vi "Process.vi"(8 "error in":errorcluster, 11 "Inst.Transport in":refnum<class "Inst.Transport.lvclass">) -> (0 "error out":errorcluster, 3 "Inst.Transport out":refnum<class "Inst.Transport.lvclass">)   [LabVIEW 2019, in "Inst.Transport.lvclass"]
doc: "---------------------------------------------------------------\nJKI State Machine Objects™\nhttp://jki.net/state-machine-objects/\nCopyright (C) 2005-2015, JKI <info@jki.net>\nALL RIGHTS RESERVED"
uses:
  Inst.Transport.lvclass
  <userlib>/LevyLab/Instrument Framework/Instrument/Instrument.lvclass
  <userlib>/LevyLab/RemoteControl/RemoteControl/Typedefs/Message--Cluster.ctl
  <userlib>/LevyLab/RemoteControl/RemoteControl/RemoteControl.lvclass
  Typedefs/PrivateEvents--MessageToProcess.ctl
  <userlib>/LevyLab/Debug/Debug.lvlib
  <vilib>/JKI/JKI SMO/SMO/SMO.lvclass
  Control Experiment/Control Experiment.lvclass
  Transport/Transport.lvclass
  <userlib>/LevyLab/Lockin-Multichannel/Instrument.DAQ/Typedefs/Sweep.Pattern--Enum.ctl
  <userlib>/LevyLab/Lockin-Multichannel/Instrument.DAQ/Instrument.DAQ.lvclass
  <userlib>/LevyLab/Lockin-Multichannel/Instrument.DAQ/Typedefs/Sweep.Channel--Cluster.ctl
  <userlib>/LevyLab/Lockin-Multichannel/Instrument.DAQ/Typedefs/Sweep.Channel--Cluster--Array.ctl
  Transport/Typedefs/Lockin_Sweep JSON--Cluster.ctl
  Typedefs/Inst.Transport.PublicCommands--Enum.ctl
  Typedefs/Inst.Transport.Methods--Enum.ctl
  Typedefs/startTransport--Request--Cluster.ctl
  <userlib>/LevyLab/Instrument Framework/Instrument/API/Instrument.sendMessageToProcess (variant).vi
  <userlib>/LevyLab/Instrument Framework/Instrument Types/SCPI/Instrument.SCPI.lvclass
  Typedefs/Inst.Transport.ProtectedCommands--Enum.ctl
  Typedefs/Inst.Transport.Status--Enum.ctl
  Typedefs/UI State--enum.ctl
  C:/Program Files (x86)/National Instruments/LabVIEW 2019/user.lib/LevyLab/Instrument Framework/Instrument Types/SCPI/Instrument.SCPI.lvclass
  C:/Program Files (x86)/National Instruments/LabVIEW 2019/user.lib/LevyLab/Instrument Framework/Instrument/Instrument.lvclass
  C:/Program Files (x86)/National Instruments/LabVIEW 2019/vi.lib/JKI/JKI SMO/SMO/SMO.lvclass
  Typedefs/RefreshTime--Request--Cluster.ctl
  db7760a1-0849-494e-b918-bfd2b1278472.vi
  48eb5b5f-56a5-4c0e-b192-c05c3e35427f.vi
  1045582e-a15c-4059-9878-8d398bb7fea9.vi
  8f0a8fc2-545a-492d-a380-fe326c3f5926.vi
panel:
  in  "Tab Control":enum32{"Main", "Debug"}(tab)
  in  "stopTransport":bool
  out "Status":string
  in  "Close VI":bool
  in  "Open VI":bool
  in  "Ring":u16(ring)
  out "state history":string
  out "parameters":string
  out "command":string
  out "Secret Status":string
  # "Transport Server"
  # "Inst.Transport"
  # "For instructions on how to use the JKI State Machine Objects, examples and video tutorials, visit:\nhttp://jki.net/state-machine-objects/\n\nJKI State Machine Objects™\nhttp://jki.net/state-machine-objects/\nCopyright (C) 2005-2015, JKI <info@jki.net>\nALL RIGHTS RESERVED"
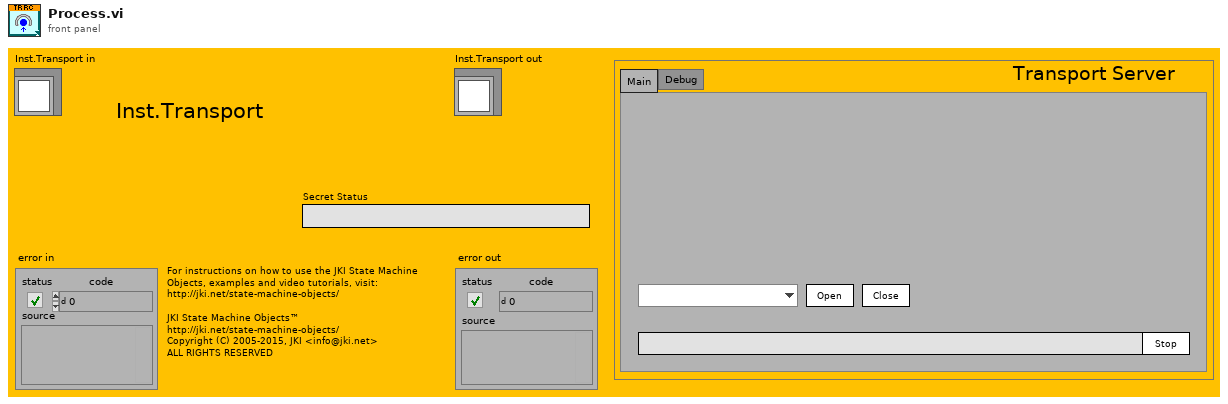
[diagram p1: front panel]
types:
  T1 = typedef "Inst.Transport.lvclass/UI State--enum.ctl" = enum16{"unknown", "Opened", "Closed"}
  T2 = typedef "Inst.Transport.lvclass/Inst.Transport.ProtectedCommands--Enum.ctl" = enum16{"setStatus", "showUI", "hideUI"}
  T3 = typedef "Inst.Transport.lvclass/Inst.Transport.PublicCommands--Enum.ctl" = enum16{"startTransport", "stopTransport", "getStatus", "setExptFolder", "getExptFolder", "setExptComments", "getExptComments", "setExptParam", "appendExptParam", "clearExptParam", "setSweepConfig", "getSweepConfig", "setRefreshTime"}
  T4 = typedef "Inst.Transport.lvclass/startTransport--Request--Cluster.ctl" = cluster{"method":T5}
  T5 = typedef "Inst.Transport.lvclass/Inst.Transport.Methods--Enum.ctl" = enum16{"LockinSweep", "LockinTime", "LockinTimeDelay"}
  T6 = enum32{"invalid app kind", "Development System", "Run Time System", "Student Edition", "Embedded LabVIEW", "Evaluation", "Custom"}
  T7 = typedef "Inst.Transport.lvclass/Inst.Transport.Status--Enum.ctl" = enum16{"idle", "running"}
  T8 = enum32{"Invalid", "Standard", "Closed", "Hidden", "Minimized", "Maximized"}
  T9 = typedef "Transport.lvclass/Lockin_Sweep JSON--Cluster.ctl" = cluster{"Sweep Time (s)":dbl, "Initial Wait (s)":dbl, "Return to Start":bool, "Sweep Channels":T10, "Sweep Tables":cluster{"Ch":i32, "Table":dbl[]}[]}
  T10 = typedef "Instrument.Lockin.lvlib/Instrument.DAQ.lvclass/Sweep.Channel--Cluster--Array.ctl" = T11[]
  T11 = typedef "Instrument.Lockin.lvlib/Instrument.DAQ.lvclass/Sweep.Channel--Cluster.ctl" = cluster{"Enable?":bool, "Channel":u16, "Start":dbl, "End":dbl, "Pattern":T12, "Table":dbl[]}
  T12 = typedef "Instrument.Lockin.lvlib/Instrument.DAQ.lvclass/Sweep.Pattern--Enum.ctl" = enum16{"Ramp /", "Ramp /\\", "Smooth Ramp _/", "Smooth Ramp _/\\_", "Table"}
  T13 = typedef "Inst.Transport.lvclass/RefreshTime--Request--Cluster.ctl" = cluster{"Refresh Time":u32}
  T14 = typedef "Inst.Transport.lvclass/PrivateEvents--MessageToProcess.ctl" = cluster{"Message":T15}
  T15 = typedef "RemoteControl.lvlib/RemoteControl.lvclass/Message--Cluster.ctl" = cluster{"Command":string, "Data":variant, "ID":string, "error":errorcluster}
  T16 = cluster{"Core":cluster{"Current VI Reference":refnum<vi>, "Close Panel on Exit?":bool, "Last Error":cluster{"error":errorcluster, "previous state":string, "remaining states":string}, "Shutdown?":bool}, "SelfRef":refnum<class "Inst.Transport.lvclass">, "Transport":refnum<class "Transport.lvclass">, "C.E.":refnum<class "Control Experiment.lvclass">, "Folder":string, "Comments":string, "notifier":refnum<notifier>, "method":T5, "paths":path[], "path":path, "Running Step":i32, "sequence":string[], "MessageToProcess":T14, "UI Behavior":string, "wait":u32}
  T17 = cluster{"Current VI Reference":refnum<vi>, "Close Panel on Exit?":bool, "Last Error":cluster{"error":errorcluster, "previous state":string, "remaining states":string}, "Shutdown?":bool}
  T18 = typedef "Debug.lvlib/Attribute.Debug.lvclass/DebugBehavior.ctl" = enum16{"Normal", "Debug"}
  T19 = typedef "SMO.lvclass/Protected Events.ctl" = cluster{"StopProcesses":refnum<user-event>, "AbortProcesses":refnum<user-event>, "Config Changed":refnum<user-event>, "Dependency":refnum<user-event>}
  T20 = typedef "LV-Data.lvclass/Dictionary--cluster.ctl" = cluster{"key":string, "value":variant}
  T21 = typedef "Inst.Transport.lvclass/Inst.Transport.getAll--Cluster.ctl" = cluster{"data":variant}
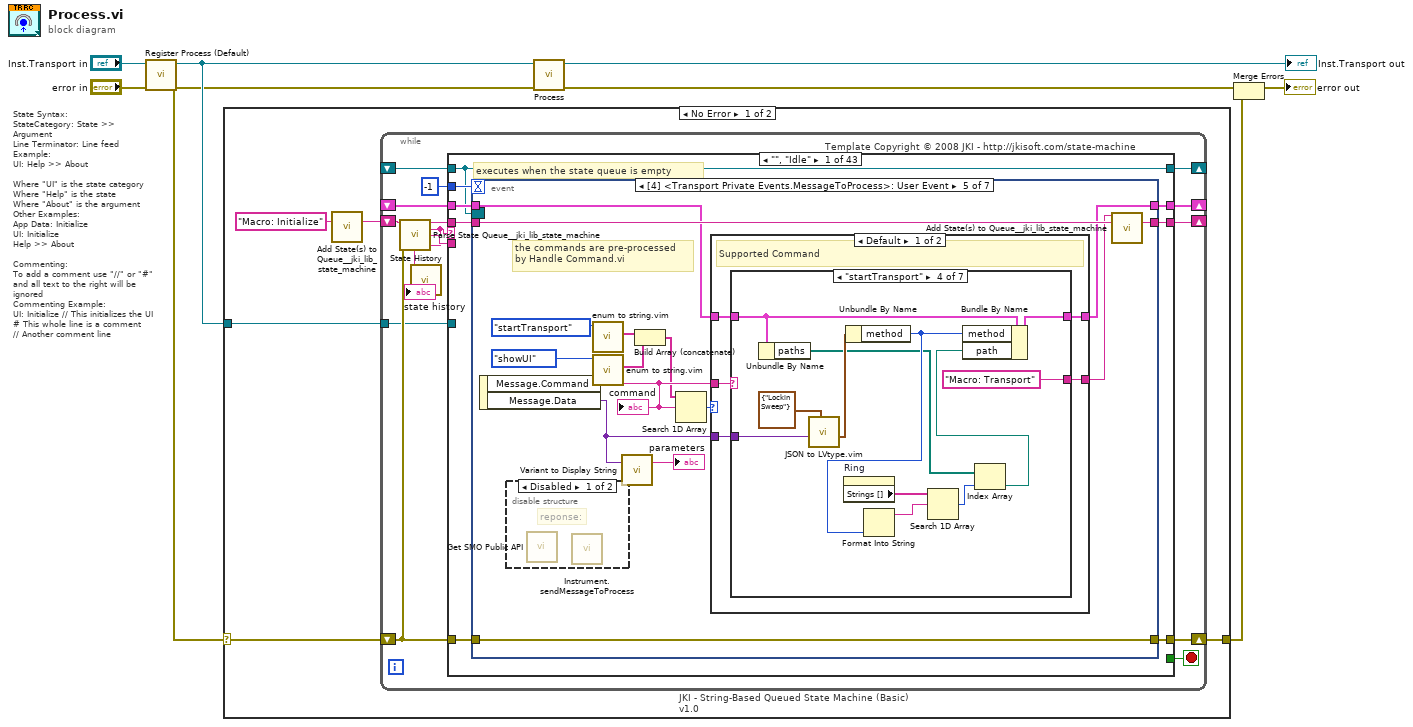
[diagram p0: block diagram]
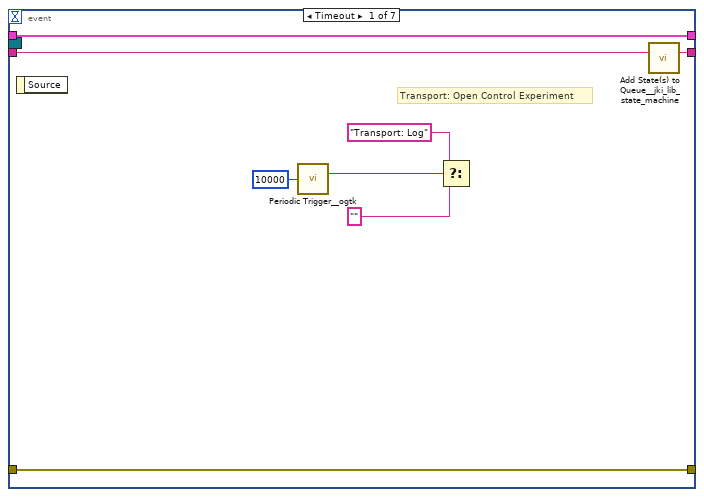
[diagram p2: hidden frame]
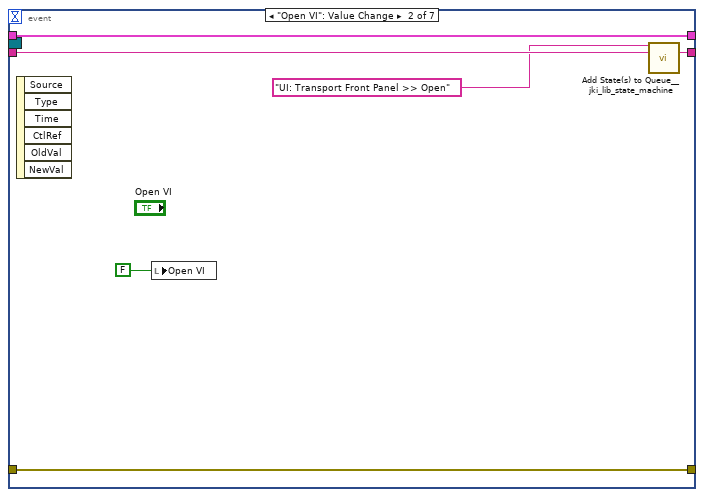
[diagram p3: hidden frame]
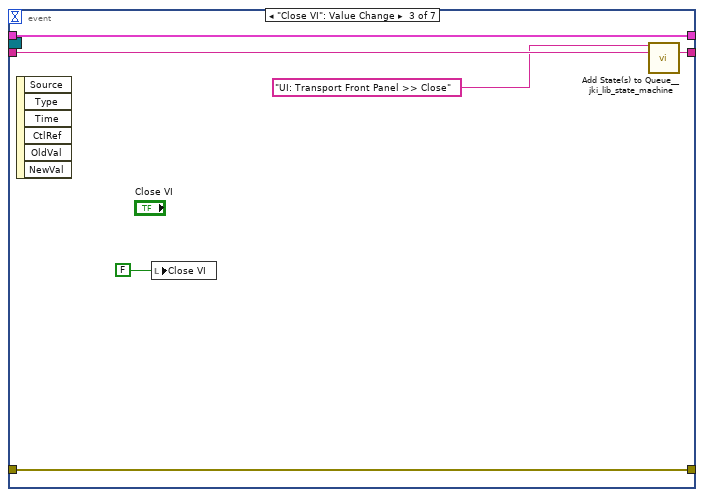
[diagram p4: hidden frame]
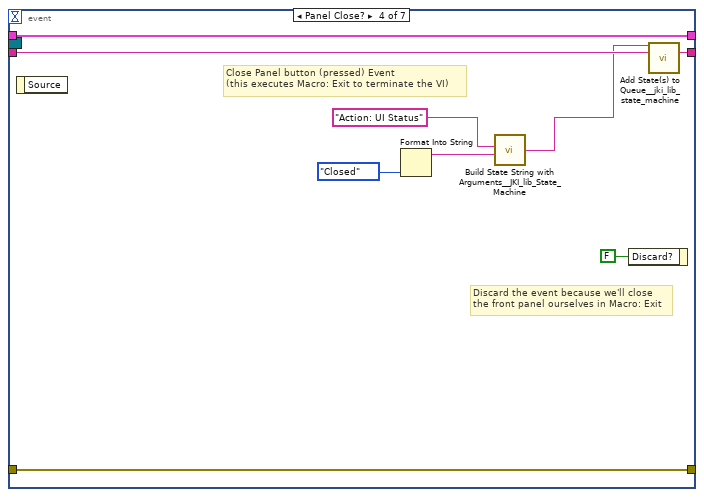
[diagram p5: hidden frame]
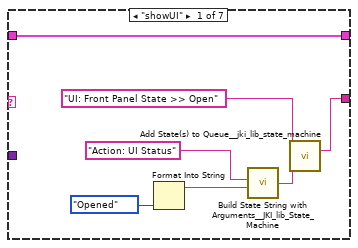
[diagram p7: hidden frame]
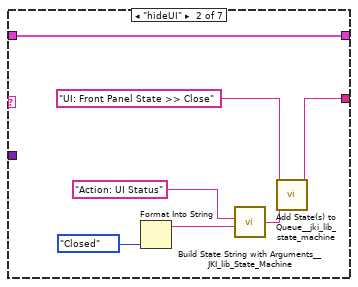
[diagram p8: hidden frame]
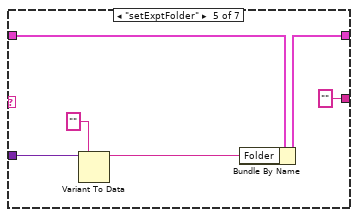
[diagram p10: hidden frame]
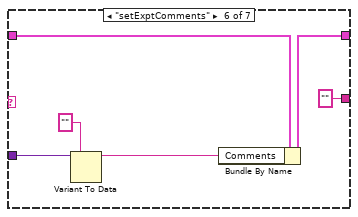
[diagram p11: hidden frame]
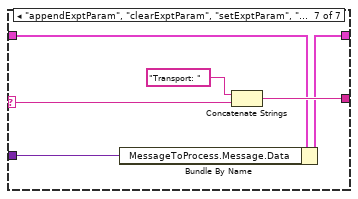
[diagram p12: hidden frame]
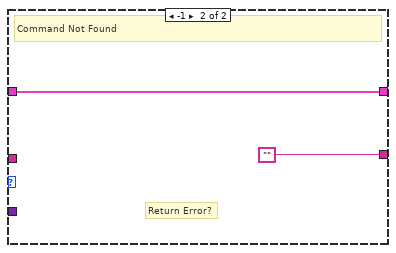
[diagram p13: hidden frame]
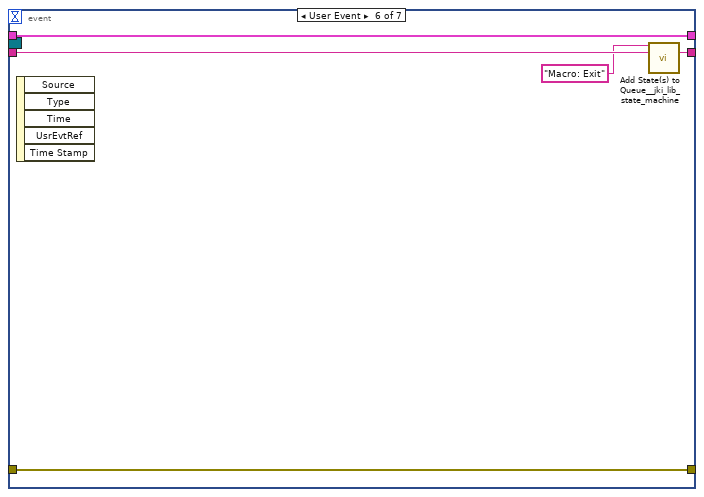
[diagram p14: hidden frame]
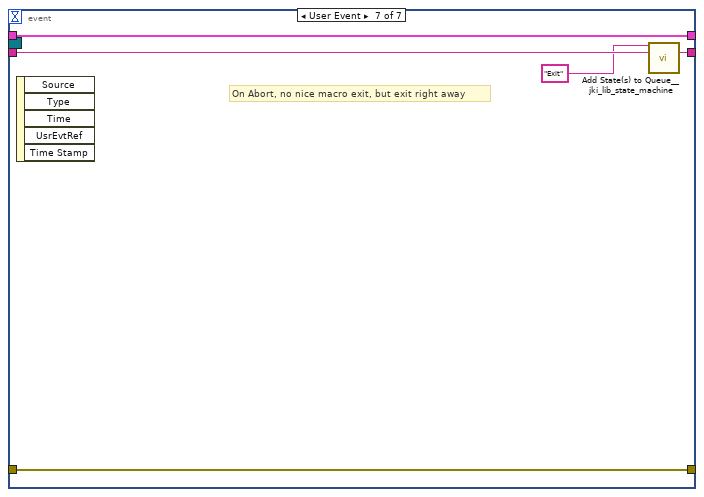
[diagram p15: hidden frame]
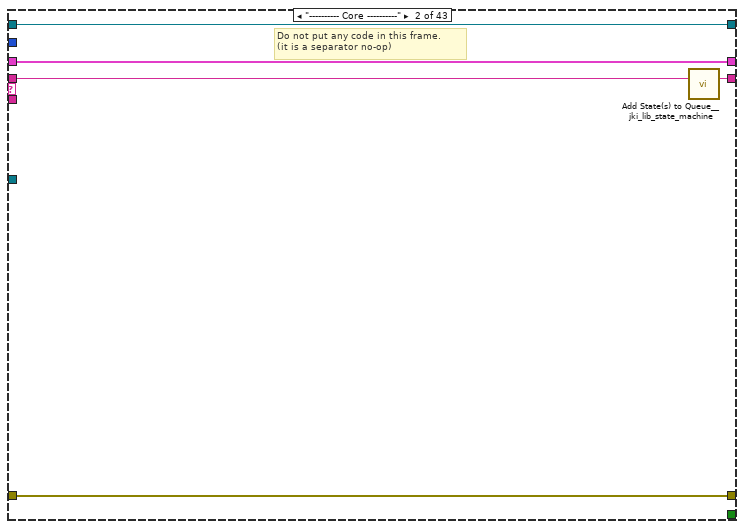
[diagram p16: hidden frame]
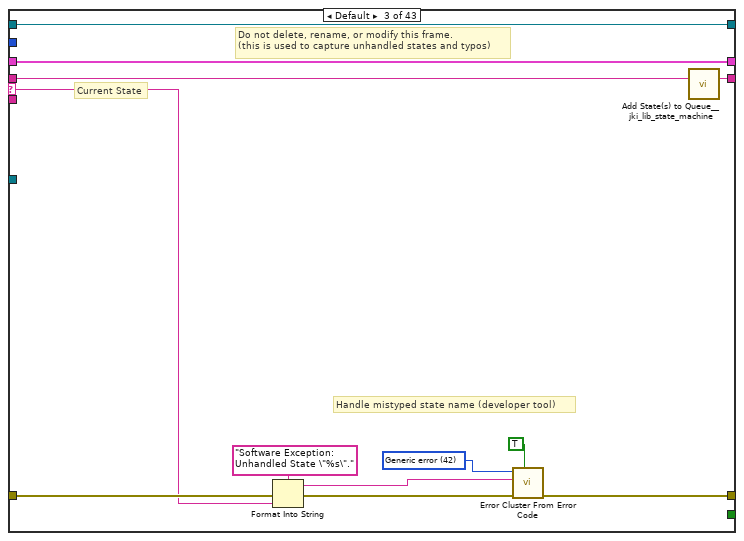
[diagram p17: hidden frame]
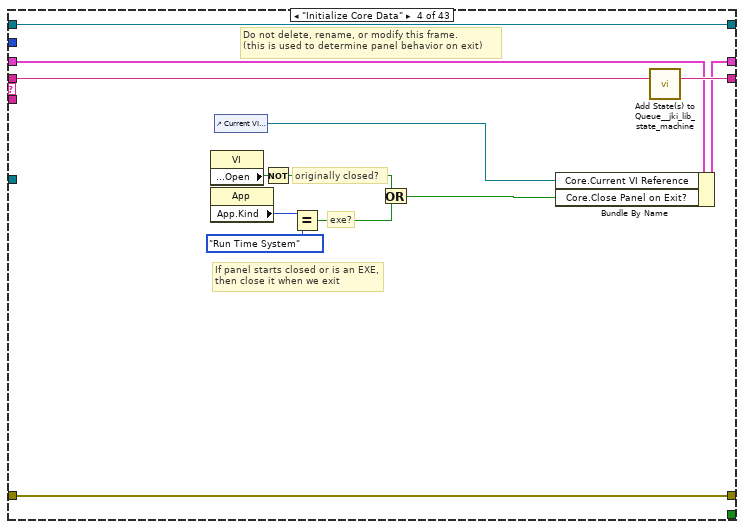
[diagram p18: hidden frame]
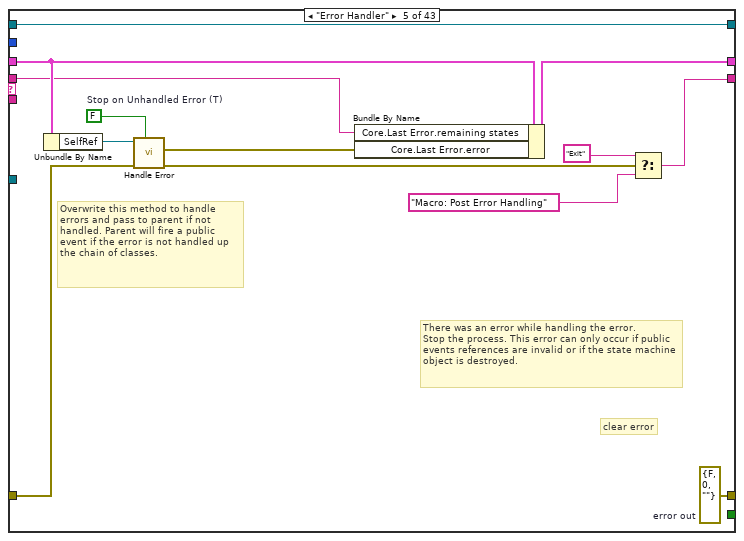
[diagram p19: hidden frame]
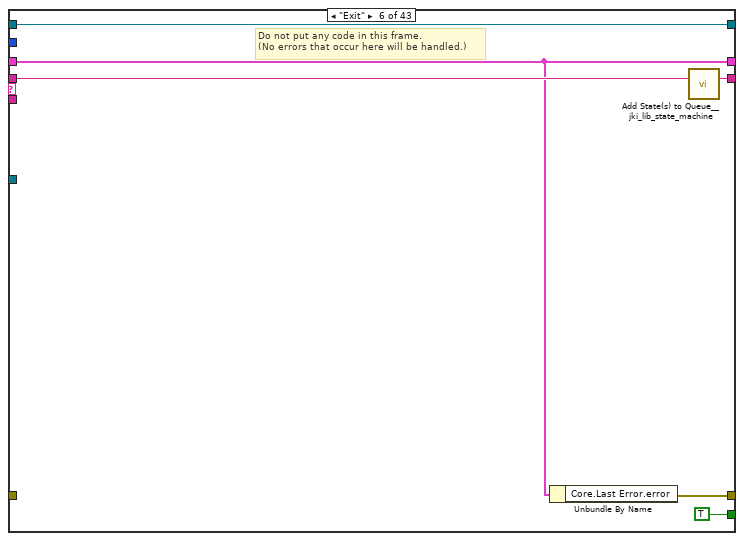
[diagram p20: hidden frame]
diagram:
  # "State Syntax:\nStateCategory: State >> Argument\nLine Terminator: Line feed\nExample:\nUI: Help >> About\n\nWhere \"UI\" is the state category\nWhere \"Help\" is the state\nWhere \"About\" is the argument\nOther Examples:\nApp Data: Initialize\nUI: Initialize\nHelp >> About\n\nCommenting:\nTo add a comment use \"//\" or \"#\" and all text to the right will be ignored\nCommenting Example:\nUI: Initialize // This initializes the UI\n# This whole line is a comment\n// Another comment line"
  n1 = call <vilib>:"Register Process (Default).vi"("error in (no error)"="error in", "SMO"="Inst.Transport in") -> ("error out"=w3:errorcluster, "SelfRef"=w6:refnum<class "Inst.Transport.lvclass">)  [unwired: 8 in]
  n2 = case shown="No Error" w3 {
    selector: w3 -> [w10 w738]
    tunnel: w6 -> [w11 _]
    tunnel: [w9 w738] -> w4
    frame No Error {
      n3 = call <vilib>:"Add State(s) to Queue__jki_lib_state_machine.vi"("State(s) in (\"\")"="Macro: Initialize") -> ("States Out"=w13:string)  [unwired: 14 in]
      n4 = while "JKI - String-Based Queued State Machine (Basic) v1.0" {
        shift-right: [w22] -> _
        shift-left: _ -> [w21]
        shift-right: [w25] -> w9
        shift-left: w10 -> [w19]
        shift-right: [w24] -> _
        shift-left: w13 -> [w26]
        tunnel: w11 -> [w18]
        shift-right: [w17] -> _
        shift-left: _ -> [w16]
        stop <- w23 stop-if-true
        # "Template Copyright © 2008 JKI - http://jkisoft.com/state-machine"
        n5 = call <vilib>:"Parse State Queue__jki_lib_state_machine.vi"("State Queue"=w26, "Error In (no error)"=w19) -> ("Remaining States"=w28:string, "Current State"=w15:string, "Arguments"=w27:string)  [unwired: 11 in]
        n6 = call <userlib>:"State History.vi"("Current State"=w15) -> ("History"=→"state history":string)  [unwired: 10 in]
        n7 = case shown="\"\", \"Idle\"" w15 {
          selector: w15 -> [_ _ w149 _ _ _ _ _ _ _ _ _ _ _ _ _ _ _ _ _ _ _ _ _ _ _ _ _ _ _ _ _ _ _ _ _ _ _ _ _ _ _ _]
          tunnel: w28 -> [w36 w147 w153 w172 w177 w191 w196 w217 w234 w263 w277 w282 w292 w301 w308 w324 w362 w404 w413 w425 w446 w461 w472 w489 w494 w505 w512 w517 w530 w536 w544 w568 w579 w636 w649 w656 w669 w683 w696 w701 w712 w718 w737]
          tunnel: w27 -> [_ _ _ _ _ _ _ _ _ w257 _ _ _ w293 w302 w318 w355 _ _ _ _ _ _ _ _ _ _ _ _ _ _ _ _ _ _ _ _ _ _ _ w705 w713 w721]
          tunnel: w21 -> [w34 w144 w151 w163 w181 w187 w193 _ w229 w260 w272 w279 w290 w298 w306 w320 w354 w401 w410 w415 w436 w450 w469 w474 w491 w502 w509 w514 w523 w534 w539 w564 w576 w632 w645 w651 w665 w679 w692 w698 w706 w714 w727]
          tunnel: [w33 w145 w155 w169 w182 w186 w194 w208 w231 w253 w273 w280 w287 w299 w303 w321 w359 w402 w405 w423 w444 w449 w470 w477 w492 w496 w507 w515 w526 w532 w541 w552 w572 w629 w642 w653 w662 w676 w690 w697 w704 w715 w729] -> w25
          tunnel: w19 -> [w32 w145 w154 w169 w183 _ w194 w208 w231 w252 w274 w280 w286 w299 w304 w322 w358 w402 w405 w423 w444 w448 w470 w477 w492 w497 w506 w515 w520 w532 w541 w554 w571 w626 w640 w653 w659 w678 w685 w697 w703 w715 w723]
          tunnel: [w35 w146 w152 w171 w173 w190 w195 w216 w233 w262 w276 w281 w291 w300 w307 w323 w361 w403 w412 w424 w445 w460 w471 w488 w493 w504 w511 w516 w529 w535 w543 w567 w578 w635 w648 w655 w668 w682 w695 w700 w711 w717 w736] -> w24
          tunnel: [_ _ _ _ _ TRUE _ _ _ _ _ _ _ _ _ _ _ _ _ _ _ _ _ _ _ _ _ _ _ _ _ _ _ _ _ _ _ _ _ _ _ _ _] -> w23
          tunnel: [w31 w144 w151 w170 w180 w187 w193 w215 w230 w260 w272 w279 w290 w298 w306 w320 w354 w401 w410 w416 w437 w451 w469 w475 w491 w502 w509 w514 w523 w534 w540 w565 w576 w633 w646 w652 w666 w680 w693 w698 w706 w714 w726] -> w22
          tunnel: -1 ("Timeout") -> [w30 _ _ _ _ _ _ _ _ _ _ _ _ _ _ _ _ _ _ _ _ _ _ _ _ _ _ _ _ _ _ _ _ _ _ _ _ _ _ _ _ _ _]
          tunnel: w18 -> [_ _ _ _ _ _ _ w209 _ _ _ _ _ _ _ _ _ _ _ _ _ _ _ _ _ _ _ _ _ _ _ _ _ _ _ _ _ _ _ _ _ _ _]
          tunnel: [w29 w143 w148 w160 w185 w188 w192 w214 w232 w261 w271 w278 w289 w297 w305 w317 w360 w400 w411 w422 w443 w459 w468 w483 w490 w503 w510 w513 w528 w533 w542 w566 w577 w634 w647 w654 w667 w681 w694 w699 w710 w716 w735] -> w17
          tunnel: w16 -> [w29 w143 w148 w160 w185 w188 w192 w214 w232 w261 w271 w278 w289 w297 w305 w317 w360 w400 w411 w422 w443 w459 w468 w483 w490 w503 w510 w513 _ w533 w542 w566 w577 w634 w647 w654 w667 w681 w694 w699 w710 w716 w735]
          frame "", "Idle" {
            # "executes when the state queue is empty"
            n8 = event shown="[4] <Transport Private Events.MessageToProcess>: User Event" {
              selector: w29 -> [_ _ _ _ _ _ _]
              dyn-events: _ -> [_ _ _ _ _ _ _]
              timeout: w30 -> [_ _ _ _ _ _ _]
              tunnel: w36 -> [w44 w50 w56 w65 w80 w137 w142]
              tunnel: [w43 w49 w55 w64 w79 w136 w141] -> w35
              tunnel: w34 -> [w41 w47 w53 w62 w74 w134 w139]
              tunnel: [w42 w48 w54 w63 w78 w135 w140] -> w33
              tunnel: w32 -> [w42 w48 w54 w63 w78 w135 w140]
              tunnel: [w41 w47 w53 w62 w73 w134 w139] -> w31
              event Timeout {
                # "Transport: Open Control Experiment"
                n9 = event-data() -> ()  [unwired: 1 in, 1 out]
                n10 = call <userlib>:"Periodic Trigger__ogtk.vi"("time (ms)"=u32 10000) -> ("Triggered"=w39:bool)  [unwired: 12 in, 2 out]
                n11 = Select(t="Transport: Log", s=w39, f="") -> ()  [unwired: 1 out]
                n12 = call <vilib>:"Add State(s) to Queue__jki_lib_state_machine.vi"("State(s) in (\"\")"=w44) -> ("States Out"=w43:string)  [unwired: 14 in]
              }
              event "Open VI": Value Change {
                n13 = event-data() -> ()  [unwired: 1 in, 6 out]
                n14 = local write "Open VI"(FALSE ("Open VI")) -> ()
                n15 = call <vilib>:"Add State(s) to Queue__jki_lib_state_machine.vi"("State(s) in Front (\"\")"="UI: Transport Front Panel >> Open" ("State(s) in Front (\"\")"), "State(s) in (\"\")"=w50) -> ("States Out"=w49:string)  [unwired: 13 in]
              }
              event "Close VI": Value Change {
                n16 = event-data() -> ()  [unwired: 1 in, 6 out]
                n17 = local write "Close VI"(FALSE ("Open VI")) -> ()
                n18 = call <vilib>:"Add State(s) to Queue__jki_lib_state_machine.vi"("State(s) in Front (\"\")"="UI: Transport Front Panel >> Close" ("State(s) in Front (\"\")"), "State(s) in (\"\")"=w56) -> ("States Out"=w55:string)  [unwired: 13 in]
              }
              event Panel Close? {
                # "Discard the event because we'll close the front panel ourselves in Macro: Exit"
                # "Close Panel button (pressed) Event\n(this executes Macro: Exit to terminate the VI)"
                n19 = event-data() -> ()  [unwired: 1 in, 1 out]
                n20 = Format Into String(UI_State--enum."Closed" ("UI State")) -> (resulting string=w57:string)  [unwired: 3 in, 1 out]
                n21 = call <vilib>:"Build State String with Arguments__JKI_lib_State_Machine.vi"("Arguments (\"\")"=w57, "State"="Action: UI Status" ("f")) -> ("State with Arguments"=w59:string)  [unwired: 4 in]
                n22 = event-data("Discard?"=FALSE) -> ()  [unwired: 1 in, 1 out]
                n23 = call <vilib>:"Add State(s) to Queue__jki_lib_state_machine.vi"("State(s) in Front (\"\")"=w59, "State(s) in (\"\")"=w65) -> ("States Out"=w64:string)  [unwired: 13 in]
              }
              event User Event {
                # "the commands are pre-processed\nby Handle Command.vi"
                n24 = event-data() -> ("Message.Command"=w72:string, "Message.Data"=w70:variant)  [unwired: 1 in]
                "command" <- w72
                n25 = disable-structure shown="Disabled" {
                  frame Disabled {
                    # "reponse:"
                    n26 = call-dynamic "Get SMO Public API.vi"() -> ()  [unwired: 9 in, 3 out]
                    n27 = call-poly <userlib>:"Instrument.sendMessageToProcess.vi"() -> ()  [unwired: 10 in, 2 out]
                  }
                  frame Enabled {
                  }
                }
                n28 = call "enum to string.vim"("enum in"=Inst.Transport.PublicCommands--Enum."startTransport" ("PublicCommands")) -> ("strings out"=w67:string[])  [unwired: 9 in, 1 out]
                n29 = call "enum to string.vim"("enum in"=Inst.Transport.ProtectedCommands--Enum."showUI" ("ProtectedCommands")) -> ("strings out"=w68:string[])  [unwired: 9 in, 1 out]
                n30 = call "Variant to Display String.vi"("Variant"=w70) -> ("xml string"=→"parameters":string)  [unwired: 2 in]
                n31 = Build Array (concatenate)(w67, w68) -> (w66:string[])
                n32 = Search 1D Array(1D array=w66, element=w72) -> (index of element=w77:i32)  [unwired: 1 in]
                n33 = case shown="Default" w77 {
                  tunnel: [w85 "" ("Empty String Constant")] -> w76
                  tunnel: w72 -> [w84 _]
                  tunnel: w70 -> [w83 _]
                  tunnel: w74 -> [w82 w131]
                  tunnel: [w81 w131] -> w73
                  frame Default {
                    # "Supported Command"
                    n34 = case shown="\"startTransport\"" w84 {
                      selector: w84 -> [_ _ _ _ _ _ w129]
                      tunnel: [w86 w93 _ "Macro: Transport" "" ("State with Arguments") "" ("State with Arguments") w128] -> w85
                      tunnel: w83 -> [_ _ _ w109 w114 w121 w127]
                      tunnel: w82 -> [w92 w99 w100 w107 w118 w124 w125]
                      tunnel: [w92 w99 w100 w112 w117 w123 w126] -> w81
                      frame "showUI" {
                        n35 = Format Into String(UI_State--enum."Opened" ("UI State")) -> (resulting string=w89:string)  [unwired: 3 in, 1 out]
                        n36 = call <vilib>:"Build State String with Arguments__JKI_lib_State_Machine.vi"("Arguments (\"\")"=w89, "State"="Action: UI Status" ("f")) -> ("State with Arguments"=w88:string)  [unwired: 4 in]
                        n37 = call <vilib>:"Add State(s) to Queue__jki_lib_state_machine.vi"("State(s) in Front (\"\")"="UI: Front Panel State >> Open" ("State with Arguments"), "State(s) at Back (\"\")"=w88) -> ("States Out"=w86:string)  [unwired: 13 in]
                      }
                      frame "hideUI" {
                        n38 = Format Into String(UI_State--enum."Closed" ("UI State")) -> (resulting string=w96:string)  [unwired: 3 in, 1 out]
                        n39 = call <vilib>:"Build State String with Arguments__JKI_lib_State_Machine.vi"("Arguments (\"\")"=w96, "State"="Action: UI Status" ("f")) -> ("State with Arguments"=w95:string)  [unwired: 4 in]
                        n40 = call <vilib>:"Add State(s) to Queue__jki_lib_state_machine.vi"("State(s) in Front (\"\")"="UI: Front Panel State >> Close" ("State with Arguments"), "State(s) at Back (\"\")"=w95) -> ("States Out"=w93:string)  [unwired: 13 in]
                      }
                      frame Default {
                      }
                      frame "startTransport" {
                        n41 = Unbundle By Name(w107) -> ("paths"=w103:path[])
                        n42 = call "JSON to LVtype.vim"("type"=T4 {"method"=enum."LockinSweep"} ("startTransport"), "JSON Data in"=w109) -> ("Data out"=w110:T4)  [unwired: 8 in, 1 out]
                        n43 = property on="Ring" class="Ring (strict)"() -> ("Strings []"=w106:string[])  [unwired: 2 in, 2 out]
                        n44 = Unbundle By Name(w110) -> ("method"=w104:T5)
                        n45 = Format Into String(w104) -> (resulting string=w105:string)  [unwired: 3 in, 1 out]
                        n46 = Search 1D Array(1D array=w106, element=w105) -> (index of element=w102:i32)  [unwired: 1 in]
                        n47 = Index Array(array=w103, index=w102) -> (element=w101:path)
                        n48 = Bundle By Name(cluster=w107, "method"=w104, "path"=w101) -> (w112:T16)
                      }
                      frame "setExptFolder" {
                        n49 = Variant To Data(type="", Variant=w114) -> (data=w113:string)  [unwired: 1 in, 1 out]
                        n50 = Bundle By Name(cluster=w118, "Folder"=w113) -> (w117:T16)
                      }
                      frame "setExptComments" {
                        n51 = Variant To Data(type="", Variant=w121) -> (data=w119:string)  [unwired: 1 in, 1 out]
                        n52 = Bundle By Name(cluster=w124, "Comments"=w119) -> (w123:T16)
                      }
                      frame "appendExptParam", "clearExptParam", "setExptParam", "setRefreshTime", "setSweepConfig" {
                        n53 = Bundle By Name(cluster=w125, "MessageToProcess.Message.Data"=w127) -> (w126:T16)
                        n54 = Concatenate Strings("Transport: ", w129) -> (w128:string)
                      }
                    }
                  }
                  frame -1 {
                    # "Return Error?"
                    # "Command Not Found"
                  }
                }
                n55 = call <vilib>:"Add State(s) to Queue__jki_lib_state_machine.vi"("State(s) in Front (\"\")"=w76, "State(s) in (\"\")"=w80) -> ("States Out"=w79:string)  [unwired: 13 in]
              }
              event User Event {
                n56 = event-data() -> ()  [unwired: 1 in, 5 out]
                n57 = call <vilib>:"Add State(s) to Queue__jki_lib_state_machine.vi"("State(s) in Front (\"\")"="Macro: Exit", "State(s) in (\"\")"=w137) -> ("States Out"=w136:string)  [unwired: 13 in]
              }
              event User Event {
                # "On Abort, no nice macro exit, but exit right away"
                n58 = event-data() -> ()  [unwired: 1 in, 5 out]
                n59 = call <vilib>:"Add State(s) to Queue__jki_lib_state_machine.vi"("State(s) in Front (\"\")"="Exit", "State(s) in (\"\")"=w142) -> ("States Out"=w141:string)  [unwired: 13 in]
              }
            }
          }
          frame "---------- Core ----------" {
            # "Do not put any code in this frame.\n(it is a separator no-op)"
            n60 = call <vilib>:"Add State(s) to Queue__jki_lib_state_machine.vi"("State(s) in (\"\")"=w147) -> ("States Out"=w146:string)  [unwired: 14 in]
          }
          frame Default {
            w158 = 42 items=["No error", "Argument error", "Memory is full", "Out of zone", "End of file", "File already open", "Generic file I/O error", "File not found", "File permission error", "Disk is full", "Duplicate path", "Too many files open", "System feature not enabled", "Resource file not found", "Cannot add resource", "Resource not found", "Image not found", "Image memory error", "Pen does not exist", "Config type invalid", "Config token not found", "Config parse error", "Config memory error", "Bad external code format", "Bad external code offset", "External code not present", "Null window", "Destroy window error", "Null menu", "Print aborted", "Bad print record", "Print driver error", "Windows error during printing", "Memory error during printing", "Print dialog error", "Generic print error", "Invalid device refnum", "Device not found", "Device parameter error", "Device unit error", "Cannot open device", "Device call aborted", "Generic error", "Cancelled by user", "Object ID too low", "Object ID too high", "Object not in heap", "Unknown heap", "Unknown object (invalid DefProc)", "Unknown object (DefProc not in table)", "Message out of range", "Invalid (null) method", "Unknown message", "Manager call not supported", "Bad address", "Network operation in progress", "Network operation timed out", "Connection is busy", "Network attribute not supported", "Network error", "Address in use", "System out of memory", "Connection aborted", "Connection refused", "Not connected", "Already connected", "Connection closed", "Initialization error (interapplication manager)", "Bad occurrence", "Wait on unbound occurrence handler", "Occurrence queue overflow", "Datalog type conflict", "Unused", "Unrecognized type (interapplication manager)", "Memory corrupt", "Failed to make temporary DLL", "Old CIN version", "Drag socket not found", "Failed to load drop-object", "Failed to register OLE object", "Failed to release OLE object", "Format specifier type mismatch", "Unknown format specifier", "Too few format specifiers", "Too many format specifiers", "Scan failed", "Newer CIN version", "Error converting to variant", "Runtime menu error", "Password tampered", "Variant attribute not found", "Incompatible variant data type", "Event data is not available", "Event Store is not present", "Occurrence is not found", "Event Queue is not created", "Event info is not available", "Refnum passed is NULL", "Error retrieving Class GUID", "Error retrieving CoClass GUID", "Error retrieving TypeLib GUID.", "Bad built application magic bytes.", "Specific driver is different from the specific driver associated with the Logical Name.", "There is no session opened to the class driver.", "Max Error", "MAX - Error with config objects", "MAX - Error loading configuration", "MAX - Group not supported"]
            # "Current State"
            # "Do not delete, rename, or modify this frame.\n(this is used to capture unhandled states and typos)"
            # "Handle mistyped state name (developer tool)"
            n61 = Format Into String(format string="Software Exception: Unhandled State \"%s\"." ("message"), error in=w154, w149) -> (resulting string=w157:string, error out=w156:errorcluster)  [unwired: 1 in]
            n62 = call <vilib>:"Error Cluster From Error Code.vi"("show call chain? (False)"=TRUE, "error in (no error)"=w156, "error message (\"\")"=w157, "error code (0)"=w158) -> ("error out"=w155:errorcluster)  [unwired: 5 in]
            n63 = call <vilib>:"Add State(s) to Queue__jki_lib_state_machine.vi"("State(s) in (\"\")"=w153) -> ("States Out"=w152:string)  [unwired: 14 in]
          }
          frame "Initialize Core Data" {
            # "Do not delete, rename, or modify this frame.\n(this is used to determine panel behavior on exit)"
            # "originally closed?"
            # "exe?"
            # "If panel starts closed or is an EXE, then close it when we exit"
            n64 = property class="VI"() -> ("Front Panel.Open"=w168:bool)  [unwired: 2 in, 2 out]
            n65 = property class="App"() -> ("App.Kind"=w167:T6)  [unwired: 2 in, 2 out]
            n66 = control-ref of="Current VI Reference"() -> (w161:refnum<vi>)
            n67 = Not(x=w168) -> (.not. x?=w165:bool)
            n68 = Equal?(x=w167, y=T6."Run Time System" ("Application:Kind")) -> (x = y?=w164:bool)
            n69 = Or(x=w165, y=w164) -> (x .or. y?=w162:bool)
            n70 = Bundle By Name(cluster=w163, "Core.Current VI Reference"=w161, "Core.Close Panel on Exit?"=w162) -> (w170:T16)
            n71 = call <vilib>:"Add State(s) to Queue__jki_lib_state_machine.vi"("State(s) in (\"\")"=w172) -> ("States Out"=w171:string)  [unwired: 14 in]
          }
          frame "Error Handler" {
            w178 = FALSE  # Stop on Unhandled Error (T)
            w182 = errorcluster {"status"=FALSE, "code"=0, "source"=""}  # error out
            # "clear error"
            # "There was an error while handling the error.\nStop the process. This error can only occur if public events references are invalid or if the state machine object is destroyed."
            # "Overwrite this method to handle errors and pass to parent if not handled. Parent will fire a public event if the error is not handled up the chain of classes."
            n72 = Unbundle By Name(w181) -> ("SelfRef"=w184:refnum<class "Inst.Transport.lvclass">)
            n73 = call-dynamic "Handle Error.vi"("Stop on Unhandled Error (T)"=w178, "error in"=w183, "SMO"=w184) -> ("handling error"=w174:errorcluster, "Unhandled error"=w179:errorcluster)  [unwired: 6 in, 1 out]
            n74 = Bundle By Name(cluster=w181, "Core.Last Error.remaining states"=w177, "Core.Last Error.error"=w179) -> (w180:T16)
            n75 = Select(t="Exit", s=w174, f="Macro: Post Error Handling") -> (s? t:f=w173:string)
          }
          frame "Exit" {
            # "Do not put any code in this frame.\n(No errors that occur here will be handled.)"
            n76 = Unbundle By Name(w187) -> ("Core.Last Error.error"=w186:errorcluster)
            n77 = call <vilib>:"Add State(s) to Queue__jki_lib_state_machine.vi"("State(s) in (\"\")"=w191) -> ("States Out"=w190:string)  [unwired: 14 in]
          }
          frame "---------- Data ----------" {
            # "Do not put any code in this frame.\n(It is a separator no-op. You can make a copy of this frame to create a new Data frame)"
            n78 = call <vilib>:"Add State(s) to Queue__jki_lib_state_machine.vi"("State(s) in (\"\")"=w196) -> ("States Out"=w195:string)  [unwired: 14 in]
          }
          frame "Data: Initialize" {
            w197 = path ""  # path
            w198 = path[] []  # paths
            w199 = Inst.Transport.Methods--Enum."LockinSweep"  # method
            w206 = u32 0  # wait
            w207 = ""  # UI Behavior
            w210 = T14 {"Message"={"Command"="", "Data"=variant(string ""), "ID"="", "error"={"status"=FALSE, "code"=0, "source"=""}}}  # MessageToProcess
            w211 = string[] []  # sequence
            w212 = -1  # Running Step
            w213 = T17 {"Current VI Reference"=refnum, "Close Panel on Exit?"=FALSE, "Last Error"={"error"={"status"=FALSE, "code"=0, "source"=""}, "previous state"="", "remaining states"=""}, "Shutdown?"=FALSE}  # Core
            # "do not delete - used by framework"
            # "Initialize the shift-register data, here.\n(data names are defined by what you wire into the bundle function)"
            n79 = Unbundle By Name(w209) -> ("Transport"=w200:refnum<class "Transport.lvclass">, "Folder"=w202:string, "Comments"=w201:string, "notifier"=w205:refnum<notifier>)
            n80 = call "Read Dependencies.vi"("Transport"=w200) -> ("C.E."=w203:refnum<class "Control Experiment.lvclass">, "Transport"=w204:refnum<class "Transport.lvclass">)  [unwired: 8 in, 1 out]
            n81 = Bundle("Core"=w213, "SelfRef"=w209, "Transport"=w204, "C.E."=w203, "Folder"=w202, "Comments"=w201, "notifier"=w205, "method"=w199, "paths"=w198, "path"=w197, "Running Step"=w212, "sequence"=w211, "MessageToProcess"=w210, "UI Behavior"=w207, "wait"=w206) -> (w215:T16)  [unwired: 1 in]
            n82 = call <vilib>:"Add State(s) to Queue__jki_lib_state_machine.vi"("State(s) in (\"\")"=w217) -> ("States Out"=w216:string)  [unwired: 14 in]
          }
          frame "Data: Populate Ring" {
            n83 = Unbundle By Name(w229) -> ("SelfRef"=w227:refnum<class "Inst.Transport.lvclass">, "Transport"=w228:refnum<class "Transport.lvclass">)
            n84 = call "Application user.lib.vi"() -> ("path out"=w219:path)  [unwired: 10 in, 1 out]
            n85 = call <vilib>:"Delimited String to 1D String Array.vi"("delimiter"="\n" ("delimiter (Tab)"), "delimited string"="Lockin_time.vi\nLockin_sweep.vi\nTHz_TimeDelay.vi\nSweep Control.vi\nContinuous B Sweep.vi") -> ("string array"=w223:string[])  [unwired: 9 in]
            n86 = call <vilib>:"Delimited String to 1D String Array.vi"("delimiter"="\n" ("delimiter (Tab)"), "delimited string"="LockinTime\nLockinSweep\nLockinTimeDelay\nSweep Control\nContinuous B Sweep") -> ("string array"=w221:string[])  [unwired: 9 in]
            n87 = for {
              tunnel: [w237] -> w224 mode=indexing if=w238
              tunnel: [w242] -> w225 mode=indexing if=w238
              tunnel: w221 -> [w242] mode=indexing
              tunnel: w223 -> [w241] mode=indexing
              tunnel: w219 -> [w240]
              n88 = call <vilib>:"Recursive File List.vi"("pattern"=w241, "Folder Path"=w240) -> ("All Files in Dir"=w239:path[])  [unwired: 5 in, 4 out]
              n89 = Index Array(array=w239) -> (element=w236:path)  [unwired: 1 in]
              n90 = Empty String/Path?(string/path=w236) -> (empty?=w235:bool)
              n91 = case shown="False" w235 {
                tunnel: [w245 FALSE ("file or folder exists?")] -> w238
                tunnel: [w244 w247] -> w237
                tunnel: w236 -> [w243 w247]
                frame False {
                  n92 = call <vilib>:"Check if File or Folder Exists.vi"("path"=w243) -> ("file or folder exists?"=w245:bool, "dup path"=w244:path)  [unwired: 8 in, 1 out]
                }
                frame True {
                }
              }
            }
            n93 = Bundle By Name(cluster=w229, "SelfRef"=w227, "Transport"=w228, "paths"=w224) -> (w230:T16)
            n94 = property on="Ring" class="Ring (strict)"("Strings []"=w225) -> ()  [unwired: 2 in, 2 out]
            n95 = call <vilib>:"Add State(s) to Queue__jki_lib_state_machine.vi"("State(s) in (\"\")"=w234) -> ("States Out"=w233:string)  [unwired: 14 in]
          }
          frame "Data: Set Status" {
            # "Dat: Set Status.\n()"
            n96 = Unbundle By Name(w260) -> ("SelfRef"=w255:refnum<class "Inst.Transport.lvclass">, "method"=w259:T5)
            n97 = Scan From String(input string=w257, default 1=Inst.Transport.Status--Enum."running" ("Status")) -> (output 1=w254:T7)  [unwired: 3 in, 3 out]
            n98 = case shown="\"running\"" w254 {
              selector: w254 -> [_ w267]
              tunnel: ["" w270] -> w249
              tunnel: w259 -> [_ w268]
              tunnel: [FALSE ("Visible") TRUE ("Visible")] -> w248
              frame "idle", Default {
              }
              frame "running" {
                n99 = Format Into String(format string="%s: %s", w268, w267) -> (resulting string=w270:string)  [unwired: 2 in, 1 out]
              }
            }
            n100 = property on="stopTransport" class="Bool (strict)"("Visible"=w248) -> ()  [unwired: 2 in, 2 out]
            n101 = call <vilib>:"Build State String with Arguments__JKI_lib_State_Machine.vi"("Arguments (\"\")"=w249, "State"="Action: Status") -> ("State with Arguments"=w251:string)  [unwired: 4 in]
            n102 = call-poly <userlib>:"Instrument.sendMessageToProcess.vi"("error in (no error)"=w252, "Data"=w254, "Command"=Inst.Transport.ProtectedCommands--Enum."setStatus" ("ProtectedCommands"), "Instrument"=w255) -> ("error out"=w253:errorcluster)  [unwired: 6 in, 1 out]
            n103 = call <vilib>:"Add State(s) to Queue__jki_lib_state_machine.vi"("State(s) in Front (\"\")"=w251, "State(s) in (\"\")"=w263) -> ("States Out"=w262:string)  [unwired: 13 in]
          }
          frame "Data: Cleanup" {
            # "Cleanup any data and references, here.\n(this is called automatically, by the Macro: Exit)"
            n104 = Unbundle By Name(w272) -> ("Core.Current VI Reference"=w275:refnum<vi>)
            n105 = Close Reference(reference=w275, error in (no error)=w274) -> (error out=w273:errorcluster)
            n106 = call <vilib>:"Add State(s) to Queue__jki_lib_state_machine.vi"("State(s) in (\"\")"=w277) -> ("States Out"=w276:string)  [unwired: 14 in]
          }
          frame "---------- UI ----------" {
            # "Do not put any code in this frame.\n(It is a separator no-op. You can make a copy of this frame to create a new UI frame)"
            n107 = call <vilib>:"Add State(s) to Queue__jki_lib_state_machine.vi"("State(s) in (\"\")"=w282) -> ("States Out"=w281:string)  [unwired: 14 in]
          }
          frame "UI: Initialize" {
            w284 = FALSE ("stopTransport")
            # "Initialize the User Interface, here.\n(this is called automatically, by the Macro: Init)"
            n108 = call <userlib>:"Fit VI window to Largest Dec__ogtk.vi"("error in (no error)"=w286, "border spacing (2 px)"=0) -> ("error out"=w287:errorcluster)  [unwired: 4 in, 1 out]
            n109 = local write "Open VI"(w284) -> ()
            n110 = local write "stopTransport"(w284) -> ()
            n111 = property on="stopTransport" class="Bool (strict)"("Visible"=w284) -> ()  [unwired: 2 in, 2 out]
            n112 = local write "Tab Control"(enum32{"Main", "Debug"}."Main" ("Tab Control")) -> ()
            n113 = property on="Ring" class="Ring (strict)"("Strings []"=string[] []) -> ()  [unwired: 2 in, 2 out]
            n114 = call <vilib>:"Add State(s) to Queue__jki_lib_state_machine.vi"("State(s) in (\"\")"=w292) -> ("States Out"=w291:string)  [unwired: 14 in]
          }
          frame "UI: Wait" {
            # "Do not put any code in this frame.\n(It is a separator no-op. You can make a copy of this frame to create a new UI frame)"
            n115 = Scan From String(format string="%d", input string=w293, default 1=u32 0 ("default value 1")) -> (output 1=w294:u32)  [unwired: 2 in, 3 out]
            n116 = Wait (ms)(milliseconds to wait=w294) -> ()  [unwired: 1 out]
            n117 = call <vilib>:"Add State(s) to Queue__jki_lib_state_machine.vi"("State(s) in (\"\")"=w301) -> ("States Out"=w300:string)  [unwired: 14 in]
          }
          frame "UI: Cursor Set" {
            # "Argument"
            # "Initialize the User Interface, here.\n(this is called automatically, by the Macro: Init)"
            n118 = disable-structure shown="Default" {
              disable-tunnel: w304 -> [w309 w312]
              disable-tunnel: [w309 w311] -> w303
              disable-tunnel: w302 -> [_ w310]
              frame condition #0 {
              }
              frame condition #1 (active) {
                n119 = case shown="\"Idle\", Default" w310 {
                  tunnel: w312 -> [w314 w316]
                  tunnel: [w313 w315] -> w311
                  frame "Idle", Default {
                    n120 = call <vilib>:"Unset Busy.vi"("error in (no error)"=w314) -> ("error out"=w313:errorcluster)  [unwired: 10 in]
                  }
                  frame "Busy" {
                    n121 = call <vilib>:"Set Busy.vi"("error in (no error)"=w316) -> ("error out"=w315:errorcluster)  [unwired: 9 in, 1 out]
                  }
                }
              }
            }
            n122 = call <vilib>:"Add State(s) to Queue__jki_lib_state_machine.vi"("State(s) in (\"\")"=w308) -> ("States Out"=w307:string)  [unwired: 14 in]
          }
          frame "UI: Front Panel State" {
            # "Argument"
            # "Set Front Panel Open or Closed\n(Usage: \"UI: Front Panel State >> Open|Close\")"
            n123 = Unbundle By Name(w320) -> ("Core.Current VI Reference"=w319:refnum<vi>)
            n124 = disable-structure shown="Default" {
              disable-tunnel: w322 -> [w328 w351]
              disable-tunnel: [w327 w351] -> w321
              disable-tunnel: w319 -> [w326 _]
              disable-tunnel: w318 -> [w325 _]
              frame condition #0 (active) {
                n125 = case shown="\"Open\", Default" w325 {
                  tunnel: w328 -> [w332 w345]
                  tunnel: [w334 w346] -> w327
                  tunnel: w326 -> [w333 w343]
                  frame "Open", Default {
                    n126 = property class="VI"(reference=w333, error in=w332) -> (reference out=w330:refnum<vi>, error out=w331:errorcluster, "FP.State"=w329:T8)
                    n127 = case shown="\"Closed\"" w329 {
                      tunnel: [w337 w340] -> w334
                      tunnel: w331 -> [w336 w340]
                      tunnel: w330 -> [w335 _]
                      frame "Closed" {
                        n128 = invoke class="VI" method="FP.Open"(reference=w335, error in=w336, "Activate"=TRUE, "State"=T8."Standard") -> (error out=w337:errorcluster)  [unwired: 1 in, 4 out]
                      }
                      frame Default {
                      }
                    }
                  }
                  frame "Close" {
                    n129 = property class="VI"(reference=w343, error in=w345) -> (reference out=w342:refnum<vi>, error out=w344:errorcluster, "FP.State"=w341:T8)
                    n130 = case shown="Default" w341 {
                      tunnel: [w347 w350] -> w346
                      tunnel: w344 -> [w347 w349]
                      tunnel: w342 -> [_ w348]
                      frame "Invalid", "Closed" {
                      }
                      frame Default {
                        n131 = invoke class="VI" method="FP.Close"(reference=w348, error in=w349) -> (error out=w350:errorcluster)  [unwired: 1 in, 2 out]
                      }
                    }
                  }
                }
              }
              frame condition #1 {
              }
            }
            n132 = call <vilib>:"Add State(s) to Queue__jki_lib_state_machine.vi"("State(s) in (\"\")"=w324) -> ("States Out"=w323:string)  [unwired: 14 in]
          }
          frame "UI: Transport Front Panel" {
            n133 = Unbundle By Name(w354) -> ("paths"=w357:path[])
            n134 = Index Array(array=w357, index="Ring") -> (element=w352:path)
            n135 = Empty String/Path?(string/path=w352) -> (empty?=w353:bool)
            n136 = case shown="False" w353 {
              tunnel: [w370 w399] -> w359
              tunnel: w358 -> [w369 w399]
              tunnel: w355 -> [w368 _]
              tunnel: w352 -> [w363 _]
              frame False {
                n137 = Open VI Reference(vi path=w363, error in (no error)=w369) -> (vi reference=w366:refnum<vi>, error out=w367:errorcluster)  [unwired: 4 in]
                n138 = case shown="\"Open\", Default" w368 {
                  tunnel: w367 -> [w375 w391]
                  tunnel: [w377 w392] -> w364
                  tunnel: w366 -> [w376 w389]
                  tunnel: [w371 w386] -> w365
                  frame "Open", Default {
                    n139 = property class="VI"(reference=w376, error in=w375) -> (reference out=w373:refnum<vi>, error out=w374:errorcluster, "FP.State"=w372:T8)
                    n140 = case shown="\"Invalid\"" w372 {
                      tunnel: [w381 w385] -> w377
                      tunnel: w374 -> [w380 w385]
                      tunnel: w373 -> [w379 w384]
                      tunnel: [w378 w384] -> w371
                      frame Default {
                        n141 = invoke class="VI" method="FP.Open"(reference=w379, error in=w380, "Activate"=TRUE, "State"=T8."Standard") -> (reference out=w378:refnum<vi>, error out=w381:errorcluster)  [unwired: 1 in, 3 out]
                      }
                      frame "Invalid" {
                      }
                    }
                  }
                  frame "Close" {
                    n142 = property class="VI"(reference=w389, error in=w391) -> (reference out=w388:refnum<vi>, error out=w390:errorcluster, "FP.State"=w387:T8)
                    n143 = case shown="Default" w387 {
                      tunnel: [w394 w398] -> w392
                      tunnel: w390 -> [w394 w397]
                      tunnel: w388 -> [w393 w396]
                      tunnel: [w393 w395] -> w386
                      frame "Invalid", "Closed" {
                      }
                      frame Default {
                        n144 = invoke class="VI" method="FP.Close"(reference=w396, error in=w397) -> (reference out=w395:refnum<vi>, error out=w398:errorcluster)  [unwired: 1 in, 1 out]
                      }
                    }
                  }
                }
                n145 = Close Reference(reference=w365, error in (no error)=w364) -> (error out=w370:errorcluster)
              }
              frame True {
              }
            }
            n146 = call <vilib>:"Add State(s) to Queue__jki_lib_state_machine.vi"("State(s) in (\"\")"=w362) -> ("States Out"=w361:string)  [unwired: 14 in]
          }
          frame "---------- Macro ----------" {
            # "Do not put any code in this frame.\n(It is a separator no-op. You can make a copy of this frame to create a new Macro frame)"
            n147 = call <vilib>:"Add State(s) to Queue__jki_lib_state_machine.vi"("State(s) in (\"\")"=w404) -> ("States Out"=w403:string)  [unwired: 14 in]
          }
          frame "Macro: Initialize" {
            # "Initialization Macro\n(This is called once, when the VI starts)"
            n148 = call <vilib>:"Add State(s) to Queue__jki_lib_state_machine.vi"("State(s) in Front (\"\")"="Data: Initialize\nInitialize Core Data\nEvents: Register", "State(s) in (\"\")"="Process: Sync", "State(s) at Back (\"\")"="UI: Initialize\nUI: Front Panel State >> Close\nAction: Status >> Initializing...\nMacro: Debug\nData: Populate Ring\nAction: Status") -> ("States Out"=w408:string)  [unwired: 12 in]
            n149 = call <vilib>:"Add State(s) to Queue__jki_lib_state_machine.vi"("State(s) in Front (\"\")"=w408, "State(s) in (\"\")"=w413) -> ("States Out"=w412:string)  [unwired: 13 in]
          }
          frame "Macro: Post Error Handling" {
            # "Clear Last Error?"
            n150 = Unbundle By Name(w415) -> ("Core.Last Error.remaining states"=w417:string, "Core.Shutdown?"=w418:bool)
            n151 = Unbundle By Name(w415) -> ("Core.Last Error.error"=w421:errorcluster)
            n152 = case shown="False" FALSE {
              tunnel: w421 -> [w429 _]
              tunnel: [w429 _] -> w420
              frame False {
              }
              frame True {
              }
            }
            n153 = case shown="False" w418 {
              tunnel: w417 -> [w426 w428]
              tunnel: [w426 w427] -> w414
              frame False {
                # "These are the remaining states (at the moment the error occured). States can be altered according to business logic."
                # "NOT SHUTTING DOWN"
              }
              frame True {
                # "Developer can decide to alter the states but should be aware that during the shutdown process, there are certain states that must be run for the SMO to properly shut itself (and this process) down. As such, one can add states to perform additional clean-ups, but should append the remaining state to be executed."
                # "SHUTTING DOWN"
                n154 = call <vilib>:"Add State(s) to Queue__jki_lib_state_machine.vi"("State(s) in (\"\")"=w428) -> ("States Out"=w427:string)  [unwired: 14 in]
              }
            }
            n155 = Bundle By Name(cluster=w415, "Core.Last Error.error"=w420) -> (w416:T16)
            n156 = call <vilib>:"Add State(s) to Queue__jki_lib_state_machine.vi"("State(s) in Front (\"\")"=w414, "State(s) in (\"\")"=w425) -> ("States Out"=w424:string)  [unwired: 13 in]
          }
          frame "Macro: Run Sequence" {
            # "0,1,2,3,4,"
            # "5"
            # "Do not put any code in this frame.\n(It is a separator no-op. You can make a copy of this frame to create a new Macro frame)"
            n157 = Unbundle By Name(w436) -> ("sequence"=w432:string[], "Running Step"=w430:i32)
            n158 = Array Size(array=w432) -> (size(s)=w442:i32)
            n159 = Index Array(array=w432, index=w430) -> (element=w431:string)
            n160 = Greater Or Equal?(x=w442, y=w430) -> (x >= y?=w434:bool)
            n161 = Select(t=-1 ("Running Step"), s=w434, f=w430) -> (s? t:f=w441:i32)
            n162 = Bundle By Name(cluster=w436, "Running Step"=w441) -> (w437:T16)
            n163 = Select(t="Action: Status >> ...", s=w434, f="Idle //Check Event Structure\nMacro: Run Sequence" ("State(s) at Back (\"\")")) -> (s? t:f=w433:string)
            n164 = call <vilib>:"Add State(s) to Queue__jki_lib_state_machine.vi"("State(s) in Front (\"\")"=w431, "State(s) at Back (\"\")"=w433) -> ("States Out"=w435:string)  [unwired: 13 in]
            n165 = call <vilib>:"Add State(s) to Queue__jki_lib_state_machine.vi"("State(s) in Front (\"\")"=w435, "State(s) in (\"\")"=w446) -> ("States Out"=w445:string)  [unwired: 13 in]
          }
          frame "Macro: Debug" {
            # "exe?"
            # "If pane is an EXE, then close it when we exit"
            # "Macro: Debug\n(get debug behavior, determine UI and determine shutdown behavior)"
            n166 = Unbundle By Name(w450) -> ("Core.Close Panel on Exit?"=w453:bool, "SelfRef"=w458:refnum<class "Inst.Transport.lvclass">)
            n167 = property class="App"() -> ("App.Kind"=w456:T6)  [unwired: 2 in, 2 out]
            n168 = Equal?(x=w456, y=T6."Run Time System" ("Application:Kind")) -> (x = y?=w452:bool)
            n169 = call <userlib>:"Get Debug Mode.vi"("error in (no error)"=w448, "SMO"=w458) -> ("error out"=w449:errorcluster, "Behavior"=w457:T18)  [unwired: 7 in, 1 out]
            n170 = case shown="\"Debug\"" w457 {
              tunnel: [w462 w464] -> w454
              tunnel: w453 -> [w462 _]
              tunnel: w452 -> [_ w466]
              tunnel: [_ "UI: Front Panel State >> Open\nUI: Wait >> 1000"] -> w447
              frame "Normal", Default {
                # "respect core.close"
              }
              frame "Debug" {
                # "keep panel open\nunless exe"
                n171 = Or(x=w466, y=FALSE) -> (x .or. y?=w464:bool)
              }
            }
            n172 = Bundle By Name(cluster=w450, "Core.Close Panel on Exit?"=w454) -> (w451:T16)
            n173 = call <vilib>:"Add State(s) to Queue__jki_lib_state_machine.vi"("State(s) in Front (\"\")"=w447, "State(s) in (\"\")"=w461) -> ("States Out"=w460:string)  [unwired: 13 in]
          }
          frame "Macro: Transport" {
            # "\"Macro: Transport\" \n()"
            n174 = call <vilib>:"Add State(s) to Queue__jki_lib_state_machine.vi"("State(s) in Front (\"\")"="Transport: prepareTransport\nData: Set Status >> running\nTransport: startTransport\nData: Set Status >> idle" ("State(s) in Front (\"\")"), "State(s) in (\"\")"=w472) -> ("States Out"=w471:string)  [unwired: 13 in]
          }
          frame "Macro: Exit" {
            # "Exit Macro\n(This is called once, when the VI exits)"
            n175 = Unbundle By Name(w474) -> ("Core.Close Panel on Exit?"=w487:bool)
            n176 = Select(t="UI: Front Panel State >> Close", s=w487, f="" ("Empty String Constant")) -> (s? t:f=w485:string)
            n177 = Bundle By Name(cluster=w474, "Core.Shutdown?"=TRUE) -> (w475:T16)
            n178 = call <vilib>:"Add State(s) to Queue__jki_lib_state_machine.vi"("State(s) in Front (\"\")"="Data: Cleanup\nEvents: Unregister\n//Process: Self Terminate", "State(s) in (\"\")"="Process: Sync", "State(s) at Back (\"\")"="Exit") -> ("States Out"=w480:string)  [unwired: 12 in]
            n179 = call <vilib>:"Add State(s) to Queue__jki_lib_state_machine.vi"("State(s) in Front (\"\")"="Action: Status >> Shutting down...", "State(s) in (\"\")"=w485, "State(s) at Back (\"\")"=w480) -> ("States Out"=w484:string)  [unwired: 12 in]
            n180 = call <vilib>:"Add State(s) to Queue__jki_lib_state_machine.vi"("State(s) in Front (\"\")"=w484, "State(s) in (\"\")"=w489) -> ("States Out"=w488:string)  [unwired: 13 in]
          }
          frame "---------- Process ----------" {
            # "Template Separator\n(You can make a copy of, or modify, this frame)"
            n181 = call <vilib>:"Add State(s) to Queue__jki_lib_state_machine.vi"("State(s) in (\"\")"=w494) -> ("States Out"=w493:string)  [unwired: 14 in]
          }
          frame "Process: Sync" {
            n182 = Unbundle By Name(w502) -> ("SelfRef"=w498:refnum<class "Inst.Transport.lvclass">)
            n183 = call <vilib>:"WaitOnProcessSync.vi"("error in (no error)"=w497, "SMO"=w498) -> ("error out"=w496:errorcluster, "Don't run?"=w501:bool)  [unwired: 7 in, 1 out]
            n184 = Select(t="Data: Cleanup\nEvents: Unregister\nExit", s=w501, f="" ("Empty String Constant")) -> (s? t:f=w495:string)
            n185 = call <vilib>:"Add State(s) to Queue__jki_lib_state_machine.vi"("State(s) in Front (\"\")"=w495, "State(s) in (\"\")"=w505) -> ("States Out"=w504:string)  [unwired: 13 in]
          }
          frame "Process: Self Terminate" {
            # "Template Separator\n(You can make a copy of, or modify, this frame)"
            n186 = Unbundle By Name(w509) -> ("SelfRef"=w508:refnum<class "Inst.Transport.lvclass">)
            n187 = call <vilib>:"SelfTerminate.vi"("error in (no error)"=w506, "SMO in"=w508) -> ("error out"=w507:errorcluster)  [unwired: 8 in, 1 out]
            n188 = call <vilib>:"Add State(s) to Queue__jki_lib_state_machine.vi"("State(s) in (\"\")"=w512) -> ("States Out"=w511:string)  [unwired: 14 in]
          }
          frame "---------- Events ----------" {
            # "Template Separator\n(You can make a copy of, or modify, this frame)"
            n189 = call <vilib>:"Add State(s) to Queue__jki_lib_state_machine.vi"("State(s) in (\"\")"=w517) -> ("States Out"=w516:string)  [unwired: 14 in]
          }
          frame "Events: Register" {
            n190 = Unbundle By Name(w523) -> ("SelfRef"=w524:refnum<class "Inst.Transport.lvclass">)
            n191 = call <vilib>:"GetProtectedEvents.vi"("SMO"=w524) -> ("error out"=w522:errorcluster, "SMO Protected Events"=w527:T19, "SMO out"=w521:refnum<class "Inst.Transport.lvclass">)  [unwired: 8 in]
            n192 = call "Inst.Transport.GetPrivateEvents.vi"("Inst.Transport in"=w521) -> ("error out"=w518:errorcluster, "Transport Private Events"=w519:cluster{"MessageToProcess":refnum<user-event>})  [unwired: 8 in, 1 out]
            n193 = register-events(w527, w519) -> (reference out=w528:refnum<event-registration>, error out=w525:errorcluster)  [unwired: 2 in]
            n194 = Merge Errors(w525, w518, w522, w520) -> (w526:errorcluster)
            n195 = call <vilib>:"Add State(s) to Queue__jki_lib_state_machine.vi"("State(s) in (\"\")"=w530) -> ("States Out"=w529:string)  [unwired: 14 in]
          }
          frame "Events: Unregister" {
            n196 = Unregister For Events(event registration refnum=w533, error in=w532) -> (error out=w531:errorcluster)
            n197 = call <vilib>:"Clear Errors.vi"("error in (no error)"=w531) -> ()  [unwired: 5 in, 2 out]
            n198 = call <vilib>:"Add State(s) to Queue__jki_lib_state_machine.vi"("State(s) in (\"\")"=w536) -> ("States Out"=w535:string)  [unwired: 14 in]
          }
          frame "---------- Transport ----------" {
            n199 = Unbundle By Name(w539) -> ("SelfRef"=w537:refnum<class "Inst.Transport.lvclass">, "Transport"=w538:refnum<class "Transport.lvclass">)
            n200 = Bundle By Name(cluster=w539, "SelfRef"=w537, "Transport"=w538) -> (w540:T16)
            n201 = call <vilib>:"Add State(s) to Queue__jki_lib_state_machine.vi"("State(s) in (\"\")"=w544) -> ("States Out"=w543:string)  [unwired: 14 in]
          }
          frame "Transport: prepareTransport" {
            n202 = Unbundle By Name(w564) -> ("SelfRef"=w563:refnum<class "Inst.Transport.lvclass">, "Transport"=w546:refnum<class "Transport.lvclass">, "C.E."=w548:refnum<class "Control Experiment.lvclass">, "Comments"=w550:string, "Folder"=w549:string)
            n203 = call "Control Experiment FGV.vi"("Function"=enum16{"read", "write"}."read", "error in (no error)"=w554, "Control Experiment.lvclass"=refnum<class "Control Experiment.lvclass"> refnum) -> ("error out"=w559:errorcluster, "Control Experiment.lvclass out"=w561:refnum<class "Control Experiment.lvclass">)  [unwired: 7 in]
            n204 = call "Write Experiment Folder.vi"("error in (no error)"=w559, "Experiment Folder"=w549, "Control Experiment in"=w561) -> ("error out"=w558:errorcluster, "Control Experiment out"=w560:refnum<class "Control Experiment.lvclass">)  [unwired: 7 in]
            n205 = call "Read All Dictionary Elements.vi"("Control Experiment in"=w548) -> ("Items"=w547:T20[])  [unwired: 8 in, 2 out]
            n206 = call "Write Experiment Description.vi"("error in (no error)"=w558, "Experiment Description"=w550, "Control Experiment in"=w560) -> ("error out"=w553:errorcluster, "Control Experiment out"=w557:refnum<class "Control Experiment.lvclass">)  [unwired: 7 in]
            n207 = call "Write Dictionary Elements (Loop).vi"("error in (no error)"=w553, "Data in"=w547, "Control Experiment in"=w557) -> ("error out"=w551:errorcluster, "Control Experiment out"=w556:refnum<class "Control Experiment.lvclass">)  [unwired: 7 in]
            n208 = call "Write Dependencies.vi"("error in (no error)"=w551, "Control Experiment"=w556, "Transport in"=w546) -> ("error out"=w552:errorcluster, "Transport out"=w555:refnum<class "Transport.lvclass">)  [unwired: 7 in]
            n209 = Bundle By Name(cluster=w564, "SelfRef"=w563, "Transport"=w555) -> (w565:T16)
            n210 = call <vilib>:"Add State(s) to Queue__jki_lib_state_machine.vi"("State(s) in (\"\")"=w568) -> ("States Out"=w567:string)  [unwired: 14 in]
          }
          frame "Transport: startTransport" {
            n211 = Unbundle By Name(w576) -> ("Transport"=w574:refnum<class "Transport.lvclass">, "path"=w569:path, "method"=w573:T5, "notifier"=w575:refnum<notifier>)
            n212 = Empty String/Path?(string/path=w569) -> (empty?=w570:bool)
            n213 = case shown="False" w570 {
              tunnel: w575 -> [w587 _]
              tunnel: w574 -> [w586 _]
              tunnel: w573 -> [w585 _]
              tunnel: [w584 w623] -> w572
              tunnel: w571 -> [w583 w623]
              tunnel: w569 -> [w581 _]
              frame False {
                n214 = Get Date/Time In Seconds() -> (seconds since 1Jan1904=w582:timestamp)
                n215 = while {
                  tunnel: w587 -> [w612]
                  tunnel: w586 -> [w620]
                  tunnel: w583 -> [w621]
                  tunnel: w583 -> [w615]
                  tunnel: w581 -> [w619]
                  tunnel: w585 -> [w617]
                  tunnel: [w608] -> w580
                  stop <- w622 stop-if-true
                  # "repeat until stop notifier is received"
                  n216 = call "Inst.Transport.CallByReference.vi"("error in (no error)"=w621, "VI"=w617, "vi path"=w619, "Transport"=w620) -> ("error out"=w616:errorcluster)  [unwired: 7 in]
                  n217 = Merge Errors(w616, w615) -> (w608:errorcluster)
                  n218 = Equal?(x=Inst.Transport.Methods--Enum."LockinTimeDelay" ("input 1"), y=w617) -> (x = y?=w614:bool)
                  n219 = Get Notifier Status(notifier=w612, error in (no error)=w608) -> (notifier out=w613:refnum<notifier>, current notification=w611:bool, error out=w610:errorcluster)  [unwired: 2 out]
                  n220 = Send Notification(notification=w614, notifier=w613) -> (error out=w609:errorcluster)  [unwired: 1 in, 1 out]
                  n221 = Compound Arithmetic op=OR(w609, w614, w611, w610) -> (w622:bool)
                }
                n222 = while {
                  tunnel: w587 -> [w601]
                  tunnel: w583 -> [_]
                  tunnel: w582 -> [w593]
                  stop <- w596 stop-if-true
                  n223 = Get Date/Time In Seconds() -> (seconds since 1Jan1904=w594:timestamp)
                  n224 = Subtract(x=w594, y=w593) -> (x-y=w588:dbl)
                  n225 = local read "Secret Status"() -> (w590:string)
                  n226 = case shown="True" "stopTransport" {
                    selector: "stopTransport" -> [_ w604]
                    tunnel: w601 -> [w602 w607]
                    tunnel: [w602 w606] -> w600
                    tunnel: [_ w605] -> w599
                    frame False {
                    }
                    frame True {
                      n227 = local write "stopTransport"(FALSE ("stopTransport")) -> ()
                      n228 = Send Notification(notification=w604, notifier=w607) -> (notifier out=w606:refnum<notifier>, error out=w605:errorcluster)  [unwired: 1 in]
                    }
                  }
                  n229 = Format Into String(format string=" %.3f s", initial string=w590, w588) -> (resulting string=w589:string)  [unwired: 1 in, 1 out]
                  n230 = local write "Status"(w589) -> ()
                  n231 = Get Notifier Status(notifier=w600, error in (no error)=w599) -> (current notification=w597:bool, error out=w598:errorcluster)  [unwired: 3 out]
                  n232 = Or(x=w597, y=w598) -> (x .or. y?=w596:bool)
                  n233 = Wait (ms)(milliseconds to wait=u32 100) -> ()  [unwired: 1 out]
                }
                n234 = Merge Errors(w580, w583) -> (w584:errorcluster)
              }
              frame True {
              }
            }
            n235 = call <vilib>:"Add State(s) to Queue__jki_lib_state_machine.vi"("State(s) in (\"\")"=w579) -> ("States Out"=w578:string)  [unwired: 14 in]
          }
          frame "Transport: appendExptParam" {
            n236 = Unbundle By Name(w632) -> ("C.E."=w631:refnum<class "Control Experiment.lvclass">, "MessageToProcess.Message.Data"=w624:variant)
            n237 = call "Parse ExptParam.vi"("error in (no error)"=w626, "params in"=w624) -> ("error out"=w625:errorcluster, "value"=w627:variant, "key"=w628:string)  [unwired: 7 in]
            n238 = call "Append Dictionary Element.vi"("error in (no error)"=w625, "value"=w627, "key"=w628, "Control Experiment in"=w631) -> ("error out"=w629:errorcluster, "Control Experiment out"=w630:refnum<class "Control Experiment.lvclass">)  [unwired: 6 in]
            n239 = Bundle By Name(cluster=w632, "C.E."=w630) -> (w633:T16)
            n240 = call <vilib>:"Add State(s) to Queue__jki_lib_state_machine.vi"("State(s) in (\"\")"=w636) -> ("States Out"=w635:string)  [unwired: 14 in]
          }
          frame "Transport: setExptParam" {
            n241 = Unbundle By Name(w645) -> ("C.E."=w644:refnum<class "Control Experiment.lvclass">, "MessageToProcess.Message.Data"=w641:variant)
            n242 = call "Parse ExptParam.vi"("error in (no error)"=w640, "params in"=w641) -> ("error out"=w639:errorcluster, "value"=w637:variant, "key"=w638:string)  [unwired: 7 in]
            n243 = call "Write Dictionary Element.vi"("error in (no error)"=w639, "value"=w637, "key"=w638, "Control Experiment in"=w644) -> ("error out"=w642:errorcluster, "Control Experiment out"=w643:refnum<class "Control Experiment.lvclass">)  [unwired: 6 in]
            n244 = Bundle By Name(cluster=w645, "C.E."=w643) -> (w646:T16)
            n245 = call <vilib>:"Add State(s) to Queue__jki_lib_state_machine.vi"("State(s) in (\"\")"=w649) -> ("States Out"=w648:string)  [unwired: 14 in]
          }
          frame "Transport: clearExptParam" {
            n246 = Bundle By Name(cluster=w651, "C.E."=refnum<class "Control Experiment.lvclass"> refnum) -> (w652:T16)
            n247 = call <vilib>:"Add State(s) to Queue__jki_lib_state_machine.vi"("State(s) in (\"\")"=w656) -> ("States Out"=w655:string)  [unwired: 14 in]
          }
          frame "Transport: setSweepConfig" {
            # "variant is preprocessed\nin Handle Command\n(JSON to LVtype)"
            n248 = Unbundle By Name(w665) -> ("Transport"=w663:refnum<class "Transport.lvclass">, "MessageToProcess.Message.Data"=w660:variant)
            n249 = Variant To Data(error in=w659, type=T9 {"Sweep Time (s)"=0.0, "Initial Wait (s)"=0.0, "Return to Start"=FALSE, "Sweep Channels"=[], "Sweep Tables"=[]} ("Lockin_Sweep"), Variant=w660) -> (data=w657:T9, error out=w658:errorcluster)
            n250 = call "Write Configure Sweep.vi"("error in (no error)"=w658, "Lockin_Sweep"=w657, "Transport in"=w663) -> ("error out"=w662:errorcluster, "Transport out"=w664:refnum<class "Transport.lvclass">)  [unwired: 7 in]
            n251 = Bundle By Name(cluster=w665, "Transport"=w664) -> (w666:T16)
            n252 = call <vilib>:"Add State(s) to Queue__jki_lib_state_machine.vi"("State(s) in (\"\")"=w669) -> ("States Out"=w668:string)  [unwired: 14 in]
          }
          frame "Transport: setRefreshTime" {
            n253 = Unbundle By Name(w679) -> ("Transport"=w674:refnum<class "Transport.lvclass">, "MessageToProcess.Message.Data"=w671:variant)
            n254 = call "JSON to LVtype.vim"("type"=T13 {"Refresh Time"=0} ("setRefreshTime"), "error in (no error)"=w678, "JSON Data in"=w671) -> ("error out"=w677:errorcluster, "Data out"=w670:T13)  [unwired: 7 in]
            n255 = Unbundle By Name(w670) -> ("Refresh Time"=w673:u32)
            n256 = call "Write Refresh Time.vi"("error in (no error)"=w677, "Refresh Time (ms)"=w673, "Transport in"=w674) -> ("error out"=w676:errorcluster, "Transport out"=w675:refnum<class "Transport.lvclass">)  [unwired: 7 in]
            n257 = Bundle By Name(cluster=w679, "Transport"=w675) -> (w680:T16)
            n258 = call <vilib>:"Add State(s) to Queue__jki_lib_state_machine.vi"("State(s) in (\"\")"=w683) -> ("States Out"=w682:string)  [unwired: 14 in]
          }
          frame "Transport: Log" {
            # "THIS process.vi is responsible for logging data. Logging can be triggered in the timeout (as shown in this template proces.vi's tieout case) OR it could be triggered by data changes, or any other way you can device.\n\nThe code above will log ALL data. But you have the ability to log a subset, log some items on a different schedule, etc."
            n259 = Unbundle By Name(w692) -> ("SelfRef"=w688:refnum<class "Inst.Transport.lvclass">)
            n260 = call-dynamic "Get SMO Database Paths.vi"("error in (no error)"=w685, "Inst.Transport in"=w688) -> ("error out"=w686:errorcluster, "Paths"=w689:string, "Inst.Transport out"=w684:refnum<class "Inst.Transport.lvclass">)  [unwired: 7 in]
            n261 = Unbundle By Name(w684) -> ("Data"=w687:T21)
            n262 = call <userlib>:"Instrument.logToDatabase.vi"("error in (no error)"=w686, "Data"=w687, "Paths"=w689, "Instrument"=w684) -> ("error out"=w690:errorcluster, "Instrument out"=w691:refnum<class "Inst.Transport.lvclass">)  [unwired: 6 in]
            n263 = Bundle By Name(cluster=w692, "SelfRef"=w691) -> (w693:T16)
            n264 = call <vilib>:"Add State(s) to Queue__jki_lib_state_machine.vi"("State(s) in (\"\")"=w696) -> ("States Out"=w695:string)  [unwired: 14 in]
          }
          frame "---------- Action ----------" {
            n265 = call <vilib>:"Add State(s) to Queue__jki_lib_state_machine.vi"("State(s) in (\"\")"=w701) -> ("States Out"=w700:string)  [unwired: 14 in]
          }
          frame "Action: UI Status" {
            n266 = Unbundle By Name(w706) -> ("SelfRef"=w709:refnum<class "Inst.Transport.lvclass">)
            n267 = Unbundle By Name(w709) -> ("UI State"=w708:refnum<user-event>)
            n268 = Scan From String(input string=w705, default 1=UI_State--enum."Closed" ("event data")) -> (output 1=w702:T1)  [unwired: 3 in, 3 out]
            n269 = Generate User Event(user event=w708, event data cluster=w702, error in=w703) -> (error out=w704:errorcluster)  [unwired: 1 in, 1 out]
            n270 = call <vilib>:"Add State(s) to Queue__jki_lib_state_machine.vi"("State(s) in (\"\")"=w712) -> ("States Out"=w711:string)  [unwired: 14 in]
          }
          frame "Action: Status" {
            # "Sequence: Status\n(Use this frame to pass the status to the UI, this VI's UI, etc)"
            n271 = call <vilib>:"Add State(s) to Queue__jki_lib_state_machine.vi"("State(s) in (\"\")"=w718) -> ("States Out"=w717:string)  [unwired: 14 in]
            "Secret Status" <- w713
            "Status" <- w713
          }
          frame "Action: Wait" {
            # "Sequence: Wait\n(Non-Blocking Wait)"
            # "F = repeat this state. wait\nT = go to next state. don't wait"
            n272 = Unbundle By Name(w727) -> ("Running Step"=w720:i32)
            n273 = call <userlib>:"Wait Logic.vi"("error in (no error)"=w723, "Time"=w721) -> ("error out"=w722:errorcluster, "Status String"=w719:string, "Trigger"=w724:bool)  [unwired: 6 in, 1 out]
            n274 = Increment(x=w720) -> (x+1=w734:i32)
            n275 = Select(t=w734, s=w724, f=w720) -> (s? t:f=w725:i32)
            n276 = Select(t=u32 0, s=w724, f=u32 100 ("milliseconds to wait")) -> (s? t:f=w731:u32)
            n277 = call <userlib>:"Wait (ms)__ogtk.vi"("error in (no error)"=w722, "milliseconds to wait"=w731) -> ("error out"=w729:errorcluster)  [unwired: 8 in, 1 out]
            n278 = Bundle By Name(cluster=w727, "Running Step"=w725) -> (w726:T16)
            n279 = call <vilib>:"Build State String with Arguments__JKI_lib_State_Machine.vi"("Arguments (\"\")"=w719, "State"="Action: Status") -> ("State with Arguments"=w728:string)  [unwired: 4 in]
            n280 = call <vilib>:"Add State(s) to Queue__jki_lib_state_machine.vi"("State(s) in Front (\"\")"=w728, "State(s) in (\"\")"=w737) -> ("States Out"=w736:string)  [unwired: 13 in]
          }
        }
      }
    }
    frame Error {
    }
  }
  n281 = call-parent "Process.vi"("error in"=w3, "Instrument"=w6) -> ("error out"=w5:errorcluster, "Instrument out"=→"Inst.Transport out":refnum<class "Inst.Transport.lvclass">)  [unwired: 8 in]
  n282 = Merge Errors(w5, w4) -> (→"error out":errorcluster)
